vi "002_Data Graph.vi"(11 "Queue Ref In":T1={"UI"=refnum, "Message"=refnum, "Data"=refnum, "Caller"=refnum, "Name"="相对湿度计算", "Data Path"=path "", "Class Path"=path "", "SubPanel"=refnum, "Project Name"="", "MNT"="", "Title"="", "Data Source"=refnum, "Queue List"={}, "VI"=refnum, "UE"=refnum}) -> ()   [LabVIEW 2020]
doc: "000001"
uses:
  Alin/QMH/000 Module Data Type.ctl
  Alin/QMH/Queue Message.ctl
  <vilib>/Utility/miscctls.llb/LVMapReplaceAction.ctl
  70220797-d935-4723-bcfa-58572be4f9d0.vi
  <vilib>/Utility/file.llb/Read Delimited Spreadsheet (string).vi
  <vilib>/Utility/file.llb/Write Delimited Spreadsheet (string).vi
panel:
  out "字符串":string="功率电流密度曲线"
  in  "Panel Show":bool
  in  "Hide Data":bool
  in  "Hide Lable":bool
  in  "Data Select":bool
  in  "Panel Change":bool
  in  "Array":T2(array[cluster]) {"Data" format="%#.3f"}
  in  "XY":cluster{cluster{"Time":timestamp, sgl}[]}[](graph)
  in  "滑动杆":u8(slide) scale=0.0..100.0
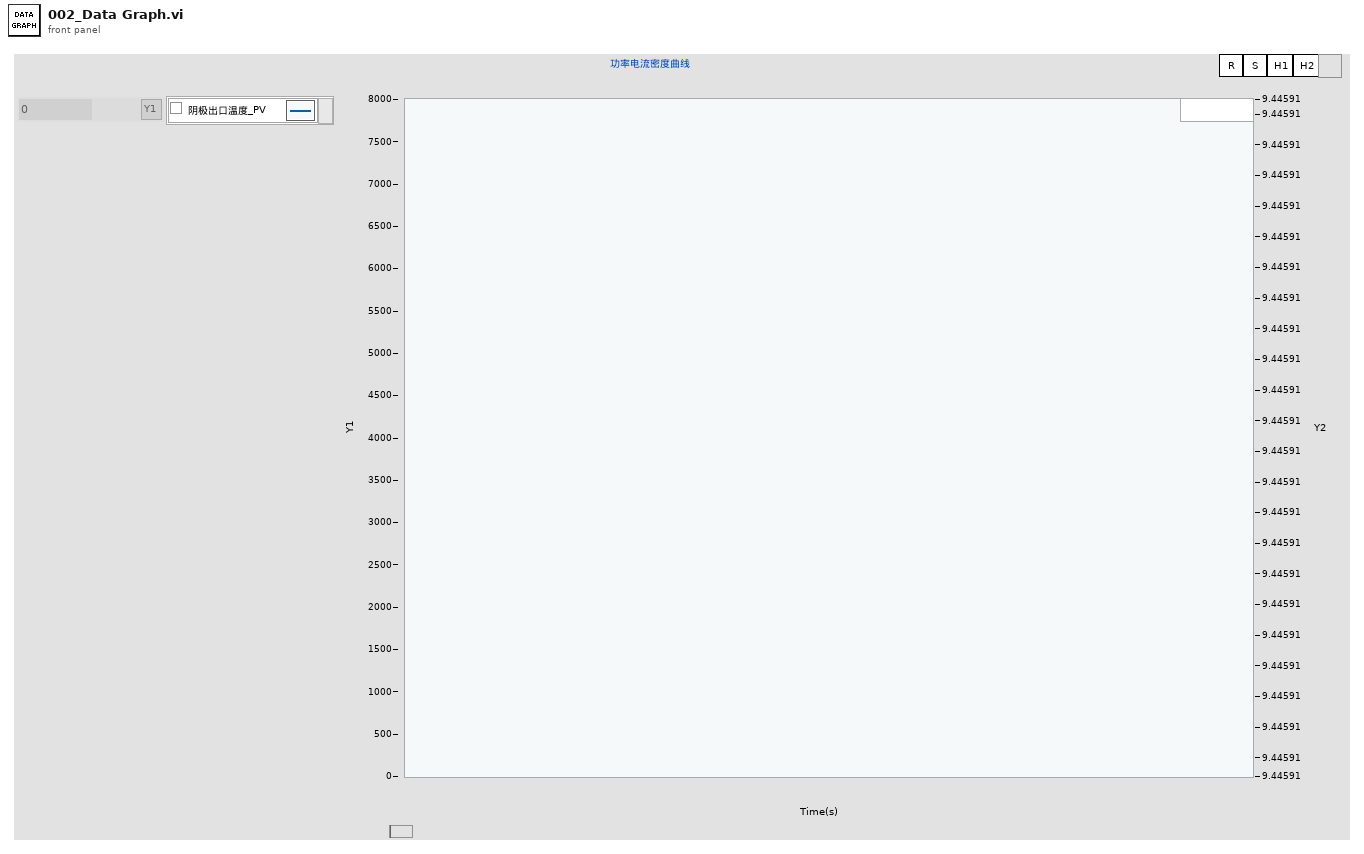
[diagram p1: front panel]
types:
  T1 = typedef "000 Module Data Type.ctl" = cluster{"UI":refnum<queue>, "Message":refnum<queue>, "Data":refnum<queue>, "Caller":refnum<queue>, "Name":string, "Data Path":path, "Class Path":path, "SubPanel":refnum<vi>, "Project Name":string, "MNT":string, "Title":string, "Data Source":refnum<queue>, "Queue List":map{string, refnum<queue>}, "VI":refnum<vi>, "UE":refnum<user-event>}
  T2 = cluster{"Identifier":string, "Data":dbl, "Unit":string, "Y":bool}[]
  T3 = cluster{"Queue Ref":T1, "Identifiers":string[], "XY":map{string, cluster{cluster{"Time":timestamp, sgl}[]}}, "Save Judge":cluster{"Time":cluster{"Name":string, "Delay":u64, "Number":u32, "Last Time":u64}[]}, "Delay":cluster{"Count Time(ms)":u32, "Delay Time(ms)":u32, "Next":string}}
  T4 = typedef "LVMapReplaceAction.ctl" = enum32{"Modify Entry only if found", "Add or Modify Entry", "Delete Entry"}
  T5 = cluster{"Name":string, "Delay":u64, "Number":u32, "Last Time":u64}[]
  T6 = cluster{"Name":string, "Delay":u64, "Number":u32, "Last Time":u64}
  T7 = typedef "SDQ Data Type.ctl" = cluster{"CAN Length":string, "CAN Name":string, "CAN ID":string, "CAN Type":string, "Test Item":string, "Byte Order":string, "Instruction":string, "Control Type":string, "Group":string, "Offset":dbl, "Coefficient":dbl, "Write Enable":bool, "Lable Type":string, "Key?":string, "Set Value":string, "Upper":dbl, "Lower":dbl, "Unit":string, "Formula":string, "Test Item Type":string, "Length":i32, "Address":string, "Name":string, "Identifier":string, "Data Type":string, "Enumerate?":string, "Enumerate List":string, "Data":string, "Source":string}
  T8 = cluster{"Identifier":string, "Data":dbl, "Unit":string, "Y":bool}
  T9 = map{string, cluster{cluster{"Time":timestamp, sgl}[]}}
  T10 = cluster{"Data Out":cluster{"Time":timestamp, sgl}[]}
  T11 = typedef "eventvkey.ctl" = enum16{"ASCII", "Enter", "Return", "Shift", "Ctrl", "Alt", "Cmd", "Opt", "Caps", "NumLock", "Clear", "Break", "Up", "Down", "Left", "Right", "Insert", "Delete", "Home", "End", "PageUp", "PageDown", "Escape", "Help", "Pause", "ScrollLock", "F1", "F2", "F3", "F4", "F5", "F6", "F7", "F8", "F9", "F10", "F11", "F12", "F13", "F14", "F15", "F16", "F17", "F18", "F19", "F20", "F21", "F22", "F23", "F24", "Play", "VolumeUp", "VolumeDown", "Mute", "Two Byte Char"}
  T12 = cluster{"Shift":bool, "Ctrl":bool, "Alt":bool, "Cmd":bool, "Opt":bool}
  T13 = typedef "LVPoint32TypeDef.ctl" = cluster{"Horizontal":i32, "Vertical":i32}
  T14 = cluster{"Queue Ref":T1, "Identifiers":string[], "XY":refnum<vi>, "Array":refnum<vi>, "Spliter":refnum<vi>}
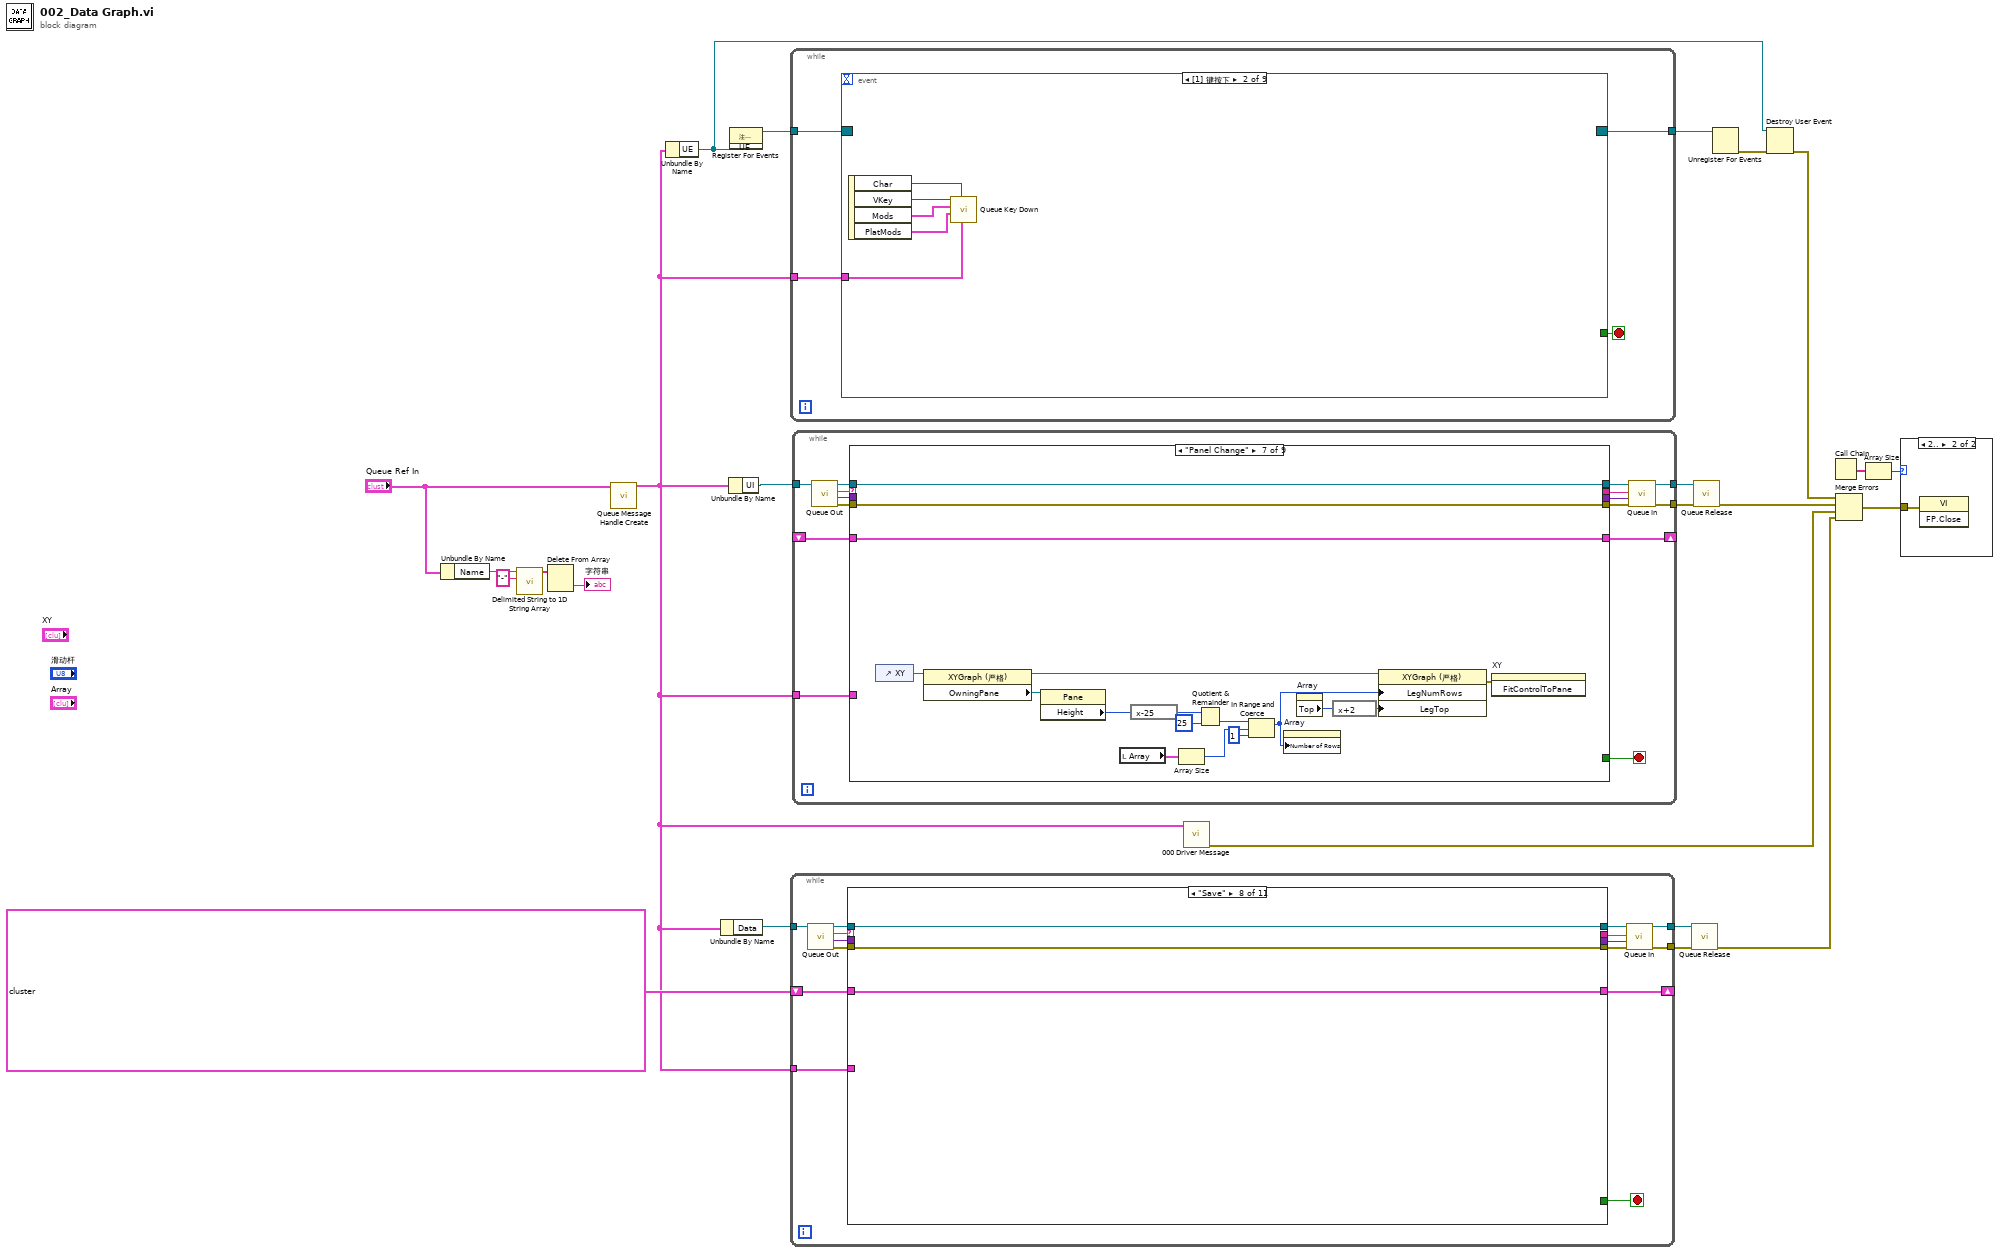
[diagram p0: block diagram]
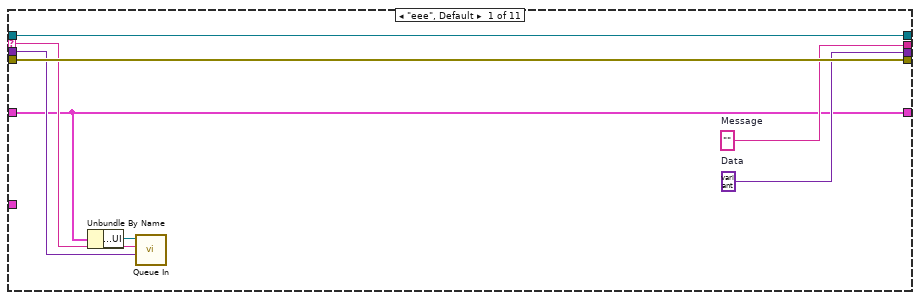
[diagram p2: hidden frame]
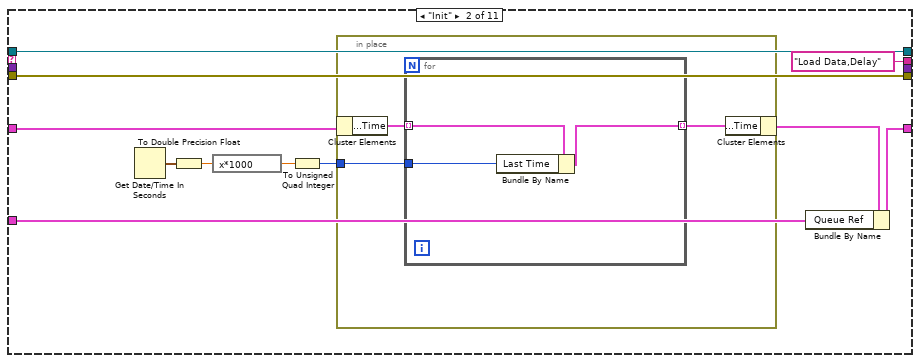
[diagram p3: hidden frame]
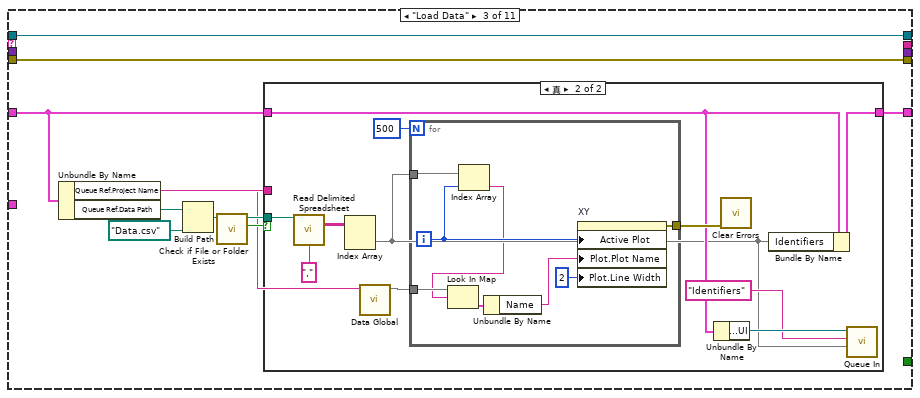
[diagram p4: hidden frame]
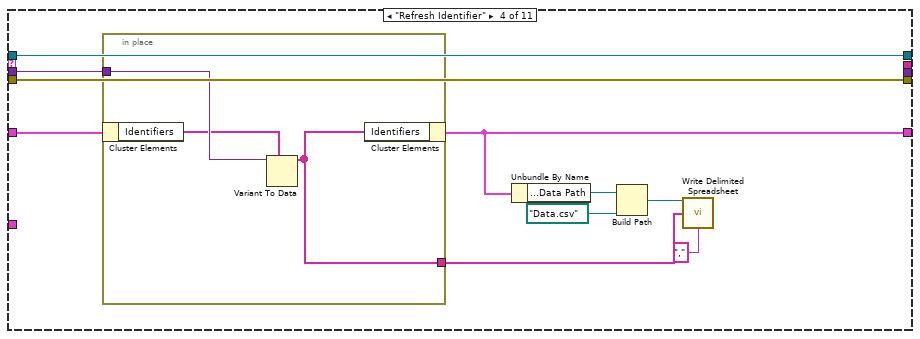
[diagram p6: hidden frame]
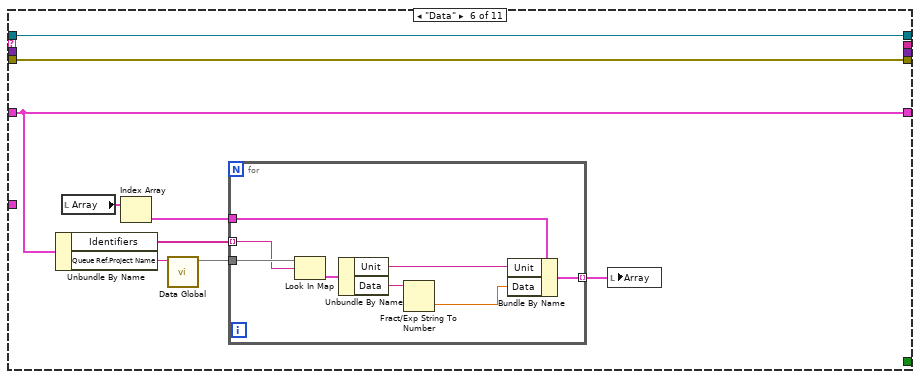
[diagram p8: hidden frame]
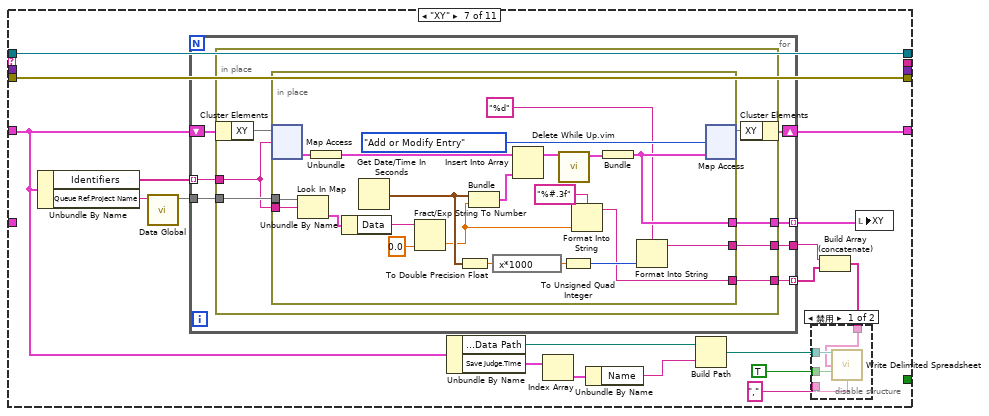
[diagram p9: hidden frame]
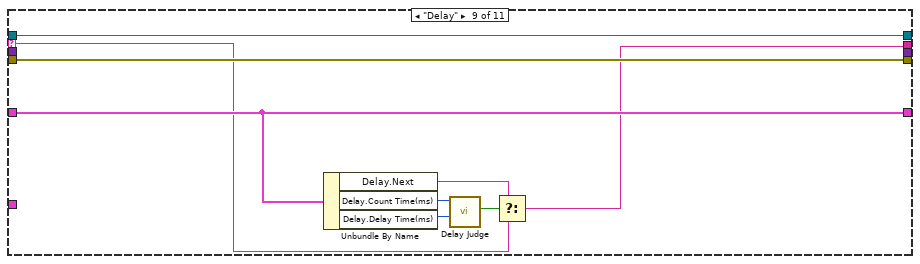
[diagram p11: hidden frame]
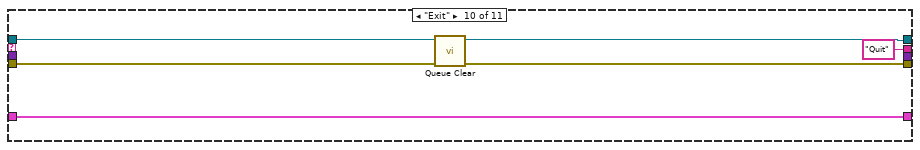
[diagram p12: hidden frame]
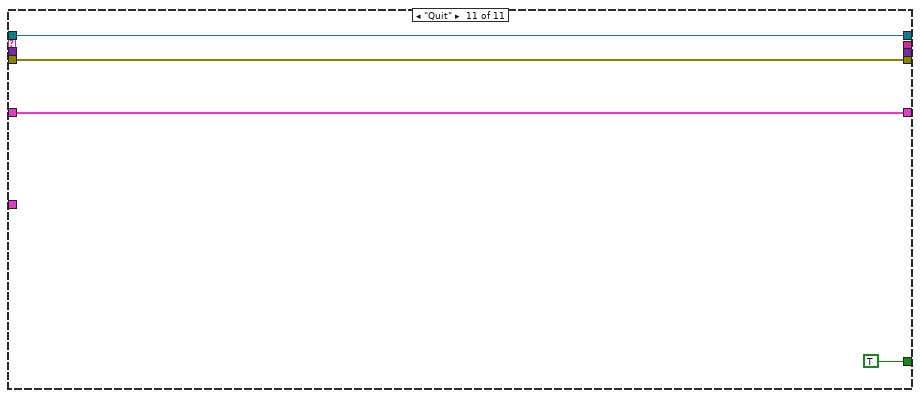
[diagram p13: hidden frame]
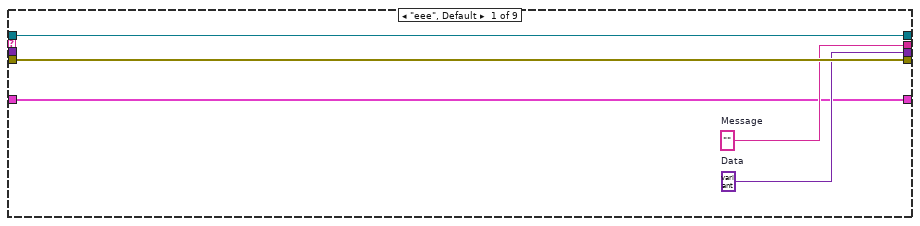
[diagram p15: hidden frame]
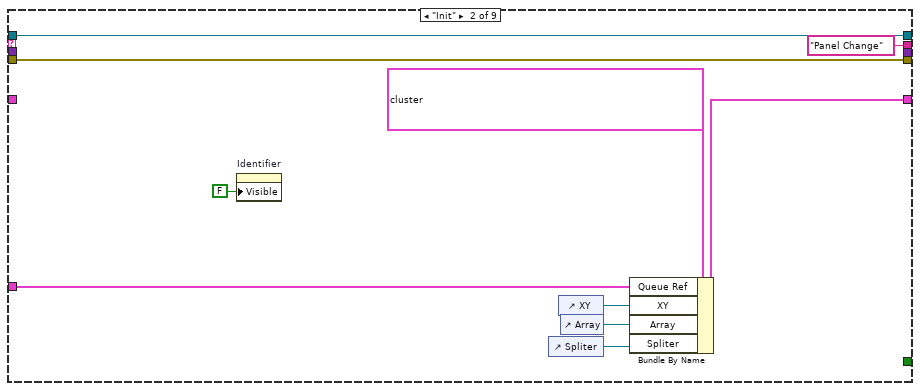
[diagram p16: hidden frame]
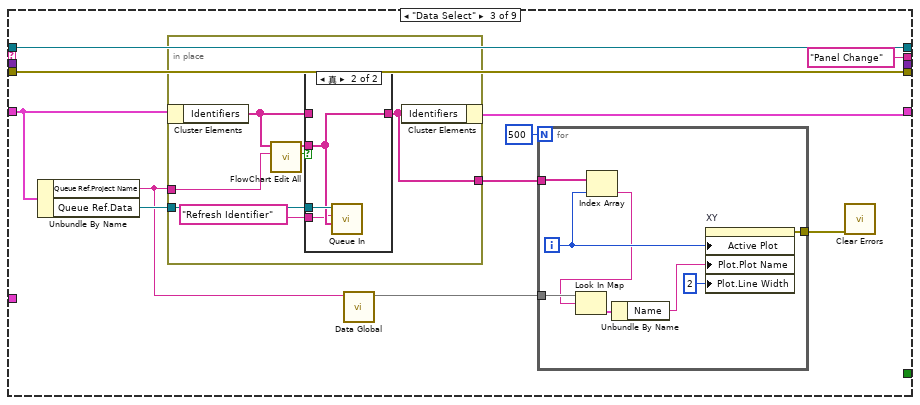
[diagram p17: hidden frame]
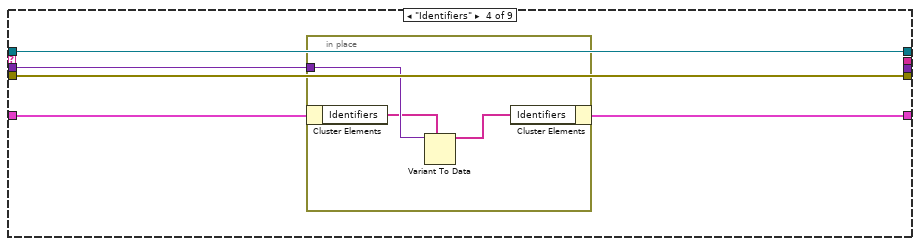
[diagram p19: hidden frame]
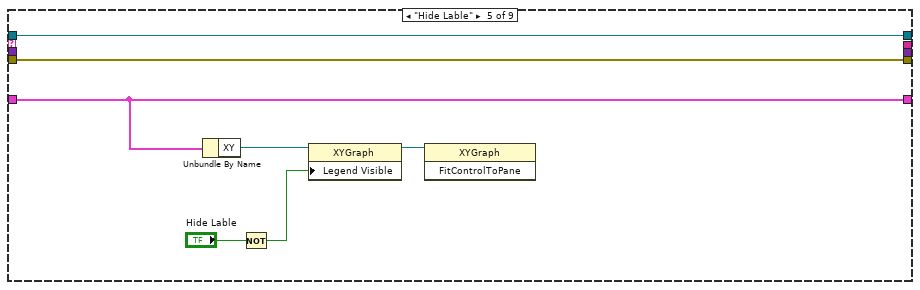
[diagram p20: hidden frame]
diagram:
  n1 = Unbundle By Name("Queue Ref In") -> ("Name"=w6:string)
  n2 = call <vilib>:"Delimited String to 1D String Array.vi"("delimiter"="-", "delimited string"=w6) -> ("string array"=w4:string[])  [unwired: 9 in]
  n3 = Delete From Array(array=w4) -> (deleted portion=→"字符串":string)  [unwired: 2 in, 1 out]
  n4 = call "Queue Message Handle Create.vi"("Queue Ref In"="Queue Ref In") -> ("Queue Ref Out"=w2:T1)  [unwired: 9 in, 1 out]
  n5 = Unbundle By Name(w2) -> ("UE"=w1:refnum<user-event>)
  n6 = Unbundle By Name(w2) -> ("Data"=w22:refnum<queue>)
  n7 = Unbundle By Name(w2) -> ("UI"=w14:refnum<queue>)
  n8 = register-events(w1) -> (reference out=w9:refnum<event-registration>)  [unwired: 2 in, 1 out]
  n9 = while {
    tunnel: w22 -> [w35]
    tunnel: [w32] -> w20
    tunnel: [w31] -> w21
    shift-right: [w27] -> _
    shift-left: T3 {"Queue Ref"={"UI"=refnum, "Message"=refnum, "Data"=refnum, "Caller"=refnum, "Name"="相对湿度计算", "Data Path"=path "", "Class Path"=path "", "SubPanel"=refnum, "Project Name"="", "MNT"="", "Title"="", "Data Source"=refnum, "Queue List"={}, "VI"=refnum, "UE"=refnum}, "Identifiers"=[], "XY"={}, "Save Judge"={"Time"=[{"Name"="Fast.csv", "Delay"=200, "Number"=0, "Last Time"=0}, {"Name"="Middle.csv", "Delay"=1000, "Number"=0, "Last Time"=0}, {"Name"="Middle.csv", "Delay"=10000, "Number"=0, "Last Time"=0}]}, "Delay"={"Count Time(ms)"=50, "Delay Time(ms)"=50, "Next"="Data,XY,Save,Delay"}} -> [w26]
    tunnel: w2 -> [w25]
    stop <- w39 stop-if-true
    n10 = call "Queue Out.vi"("Queue In"=w35) -> ("error out"=w38:errorcluster, "Data"=w36:variant, "Message"=w37:string, "Queue Out"=w34:refnum<queue>)  [unwired: 6 in, 1 out]
    n11 = case shown="\"Save\"" w37 {
      selector: w37 -> [w43 _ _ _ _ _ _ _ w190 _ _]
      tunnel: w34 -> [w47 w58 w74 w105 w111 w120 w146 w188 w197 w202 w206]
      tunnel: w38 -> [w46 w57 w73 w104 w110 w119 w145 w187 w196 w200 w207]
      tunnel: [w47 w58 w74 w105 w111 w120 w146 w188 w197 w201 w206] -> w33
      tunnel: [w46 w57 w73 w104 w110 w119 w145 w187 w196 w199 w207] -> w30
      tunnel: [w45 "Load Data,Delay" ("Message") _ _ _ _ _ _ w189 "Quit" _] -> w29
      tunnel: [_ _ _ _ _ _ _ _ _ _ TRUE] -> w39
      tunnel: [w44 _ _ _ _ _ _ _ _ _ _] -> w28
      tunnel: w36 -> [w42 _ _ w102 _ _ _ _ _ _ _]
      tunnel: [w41 w56 w67 w101 w109 w112 w144 w186 w191 w198 w204] -> w27
      tunnel: w26 -> [w41 w55 w68 w103 w109 w112 w132 w186 w191 w198 w204]
      tunnel: w25 -> [_ w48 _ _ _ _ _ _ _ _ _]
      frame "eee", Default {
        w44 = variant  # Data
        w45 = ""  # Message
        n12 = Unbundle By Name(w41) -> ("Queue Ref.UI"=w40:refnum<queue>)
        n13 = call "Queue In.vi"("Data"=w42, "Message"=w43, "Queue In"=w40) -> ()  [unwired: 7 in, 2 out]
      }
      frame "Init" {
        n14 = Get Date/Time In Seconds() -> (seconds since 1Jan1904=w53:timestamp)
        n15 = To Double Precision Float(number=w53) -> (double precision float=w52:dbl)
        n16 = expression code="x*1000"(w52) -> (w51:dbl)
        n17 = To Unsigned Quad Integer(1:w51) -> (0:w50:u64)
        n18 = in-place {
          in-place-border: w50 -> [w60]
          n19 = in-place-cluster #1(w55) -> ("Save Judge.Time"=w61:T5)
          n20 = for {
            tunnel: w61 -> [w64] mode=indexing
            tunnel: w60 -> [w63]
            tunnel: [w62] -> w59 mode=indexing
            n21 = Bundle By Name(cluster=w64, "Last Time"=w63) -> (w62:T6)
          }
          n22 = in-place-cluster #1("Save Judge.Time"=w59) -> (w54:T3)
        }
        n23 = Bundle By Name(cluster=w54, "Queue Ref"=w48) -> (w56:T3)
      }
      frame "Load Data" {
        n24 = Unbundle By Name(w68) -> ("Queue Ref.Project Name"=w65:string, "Queue Ref.Data Path"=w72:path)
        n25 = Build Path(base path=w72, name or relative path=path "Data.csv" ("名称或相对路径")) -> (appended path=w70:path)
        n26 = call <vilib>:"Check if File or Folder Exists.vi"("path"=w70) -> ("file or folder exists?"=w66:bool, "dup path"=w69:path)  [unwired: 8 in, 1 out]
        n27 = case shown="真" w66 {
          tunnel: w69 -> [_ w86]
          tunnel: w68 -> [w75 w77]
          tunnel: [w75 w84] -> w67
          tunnel: w65 -> [_ w83]
          frame False {
          }
          frame True {
            n28 = call-poly <vilib>:"Read Delimited Spreadsheet.vi"("file path (dialog if empty)"=w86, "delimiter (\\t)"="," ("delimiter (\\t)")) -> ("all rows"=w87:string[][])  [unwired: 8 in, 5 out]
            n29 = Index Array(array=w87) -> (element=w76:string[])  [unwired: 2 in]
            n30 = call "Data Global.vi"("Name"=w83) -> ("Data Out"=w82:map{string, T7})  [unwired: 7 in, 3 out]
            n31 = for {
              N: 500 -> [_]
              tunnel: [w95] -> w81
              tunnel: w82 -> [w93]
              tunnel: w76 -> [w91]
              i -> [w90]
              n32 = Index Array(array=w91, index=w90) -> (element=w89:string)
              n33 = Look In Map(map=w93, key=w89) -> (value=w94:T7)  [unwired: 1 in, 1 out]
              n34 = Unbundle By Name(w94) -> ("Name"=w92:string)
              n35 = property on="XY" class="XYGraph (严格)"("Active Plot"=w90, "Plot.Plot Name"=w92, "Plot.Line Width"=u8 2 ("曲线.线条宽度")) -> (error out=w95:errorcluster)  [unwired: 2 in, 1 out]
            }
            n36 = Unbundle By Name(w77) -> ("Queue Ref.UI"=w79:refnum<queue>)
            n37 = call <vilib>:"Clear Errors.vi"("error in (no error)"=w81) -> ()  [unwired: 5 in, 2 out]
            n38 = Bundle By Name(cluster=w77, "Identifiers"=w76) -> (w84:T3)
            n39 = call "Queue In.vi"("Data"=w76, "Message"="Identifiers", "Queue In"=w79) -> ()  [unwired: 7 in, 2 out]
          }
        }
      }
      frame "Refresh Identifier" {
        n40 = in-place {
          in-place-border: w102 -> [w108]
          in-place-border: [w106] -> w96
          n41 = in-place-cluster #2(w103) -> ("Identifiers"=w107:string[])
          n42 = Variant To Data(type=w107, Variant=w108) -> (data=w106:string[])  [unwired: 1 in, 1 out]
          n43 = in-place-cluster #2("Identifiers"=w106) -> (w101:T3)
        }
        n44 = Unbundle By Name(w101) -> ("Queue Ref.Data Path"=w100:path)
        n45 = Build Path(base path=w100, name or relative path=path "Data.csv" ("名称或相对路径")) -> (appended path=w99:path)
        n46 = call-poly <vilib>:"Write Delimited Spreadsheet.vi"("file path (dialog if empty)"=w99, "1D data"=w96, "delimiter (\\t)"="," ("delimiter (\\t)")) -> ()  [unwired: 11 in, 2 out]
      }
      frame "Data Select" {
      }
      frame "Data" {
        n47 = Unbundle By Name(w112) -> ("Identifiers"=w116:string[], "Queue Ref.Project Name"=w118:string)
        n48 = local read "Array"() -> (w115:T2)
        n49 = Index Array(array=w115) -> (element=w114:T8)  [unwired: 1 in]
        n50 = call "Data Global.vi"("Name"=w118) -> ("Data Out"=w117:map{string, T7})  [unwired: 7 in, 3 out]
        n51 = for {
          tunnel: w117 -> [w128]
          tunnel: w116 -> [w121] mode=indexing
          tunnel: w114 -> [w127]
          tunnel: [w124] -> w113 mode=indexing
          n52 = Look In Map(map=w128, key=w121) -> (value=w126:T7)  [unwired: 1 in, 1 out]
          n53 = Unbundle By Name(w126) -> ("Unit"=w125:string, "Data"=w123:string)
          n54 = Fract/Exp String To Number(string=w123) -> (number=w122:dbl)  [unwired: 3 in, 1 out]
          n55 = Bundle By Name(cluster=w127, "Unit"=w125, "Data"=w122) -> (w124:T8)
        }
        n56 = local write "Array"(w113) -> ()
      }
      frame "XY" {
        n57 = Unbundle By Name(w132) -> ("Identifiers"=w143:string[], "Queue Ref.Project Name"=w142:string)
        n58 = call "Data Global.vi"("Name"=w142) -> ("Data Out"=w141:map{string, T7})  [unwired: 7 in, 3 out]
        n59 = for {
          shift-right: [w156] -> w144
          shift-left: w132 -> [w157]
          tunnel: w143 -> [w155] mode=indexing
          tunnel: w141 -> [w154]
          tunnel: [w153] -> w140 mode=indexing
          tunnel: [w152] -> w131
          tunnel: [w151] -> w130 mode=indexing
          n60 = in-place {
            in-place-border: w155 -> [w160]
            in-place-border: w154 -> [w162]
            in-place-border: [w161] -> w153
            in-place-border: [w159] -> w152
            in-place-border: [w158] -> w151
            n61 = in-place-cluster #3(w157) -> ("XY"=w164:T9)
            n62 = in-place {
              in-place-border: w162 -> [w179]
              in-place-border: w160 -> [w177]
              in-place-border: [w176] -> w161
              in-place-border: [w168] -> w159
              in-place-border: [w167] -> w158
              n63 = in-place-map #4(w164, w160) -> (w184:cluster{cluster{"Time":timestamp, sgl}[]})  [unwired: 1 in, 1 out]
              n64 = Look In Map(map=w179, key=w177) -> (value=w181:T7)  [unwired: 1 in, 1 out]
              n65 = Unbundle(w184) -> (w183:cluster{"Time":timestamp, sgl}[])
              n66 = Unbundle By Name(w181) -> ("Data"=w180:string)
              n67 = Get Date/Time In Seconds() -> (seconds since 1Jan1904=w173:timestamp)
              n68 = Fract/Exp String To Number(string=w180, default (0 dbl)=sgl 0.0 ("默认(0 DBL)")) -> (number=w169:sgl)  [unwired: 2 in, 1 out]
              n69 = To Double Precision Float(number=w173) -> (double precision float=w175:dbl)
              n70 = Bundle("seconds since 1Jan1904"=w173, w169) -> (w182:cluster{"seconds since 1Jan1904":timestamp, sgl})  [unwired: 1 in]
              n71 = expression code="x*1000"(w175) -> (w174:dbl)
              n72 = Insert Into Array(array=w183, new element=w182) -> (w166:cluster{"Time":timestamp, sgl}[])  [unwired: 1 in]
              n73 = call "Delete While Up.vim"("Data In"=w166) -> ("Data Out"=w165:cluster{"Time":timestamp, sgl}[])  [unwired: 10 in]
              n74 = To Unsigned Quad Integer(1:w174) -> (0:w171:u64)
              n75 = Format Into String(format string="%#.3f" ("格式字符串"), w169) -> (resulting string=w167:string)  [unwired: 2 in, 1 out]
              n76 = Bundle("Data Out"=w165) -> (w176:T10)  [unwired: 1 in]
              n77 = Format Into String(format string="%d" ("格式字符串"), w171) -> (resulting string=w168:string)  [unwired: 2 in, 1 out]
              n78 = in-place-map #4(w176, LVMapReplaceAction."Add or Modify Entry" ("操作")) -> (w163:T9)  [unwired: 2 out]
            }
            n79 = in-place-cluster #3("XY"=w163) -> (w156:T3)
          }
        }
        n80 = Unbundle By Name(w132) -> ("Queue Ref.Data Path"=w137:path, "Save Judge.Time"=w139:T5)
        n81 = Index Array(array=w139) -> (element=w138:T6)  [unwired: 1 in]
        n82 = Unbundle By Name(w138) -> ("Name"=w136:string)
        n83 = Build Path(base path=w137, name or relative path=w136) -> (appended path=w135:path)
        n84 = Build Array (concatenate)(w131, w130) -> (w129:string[])
        n85 = disable-structure shown="禁用" {
          disable-tunnel: w135 -> [w150 _]
          disable-tunnel: TRUE ("append to file? (new file:F)") -> [w149 _]
          disable-tunnel: "," ("delimiter (\\t)") -> [w148 _]
          disable-tunnel: w129 -> [w147 _]
          frame Disabled {
            n86 = call-poly <vilib>:"Write Delimited Spreadsheet.vi"("file path (dialog if empty)"=w150, "1D data"=w147, "append to file? (new file:F)"=w149, "delimiter (\\t)"=w148) -> ()  [unwired: 10 in, 2 out]
          }
          frame Enabled {
          }
        }
        n87 = local write "XY"(w140) -> ()
      }
      frame "Save" {
      }
      frame "Delay" {
        n88 = Unbundle By Name(w191) -> ("Delay.Next"=w192:string, "Delay.Count Time(ms)"=w195:u32, "Delay.Delay Time(ms)"=w194:u32)
        n89 = call "Delay Judge.vi"("Delay Time(ms)"=w194, "Count Time(ms)"=w195) -> ("Time Out?"=w193:bool)  [unwired: 5 in, 4 out]
        n90 = Select(t=w192, s=w193, f=w190) -> (s? t:f=w189:string)
      }
      frame "Exit" {
        n91 = call "Queue Clear.vi"("error in (no error)"=w200, "Queue In"=w202) -> ("error out"=w199:errorcluster, "Queue Out"=w201:refnum<queue>)  [unwired: 8 in]
      }
      frame "Quit" {
      }
    }
    n92 = call "Queue In.vi"("error in (no error)"=w30, "Data"=w28, "Message"=w29, "Queue In"=w33) -> ("error out"=w31:errorcluster, "Queue Out"=w32:refnum<queue>)  [unwired: 6 in]
  }
  n93 = while {
    tunnel: w9 -> [w211]
    tunnel: [w209] -> w10
    tunnel: w2 -> [w208]
    stop <- w210 stop-if-true
    n94 = event shown="[1] 键按下" {
      selector: w211 -> [_ _ _ _ _ _ _ _ _]
      dyn-events: [_ _ _ _ _ _ _ _ _] -> w209
      timeout: _ -> [_ _ _ _ _ _ _ _ _]
      tunnel: [_ _ _ w223 _ _ _ _ _] -> w210
      tunnel: w208 -> [w214 w218 w222 _ w228 _ w242 _ w260]
      event Timeout {
        n95 = event-data() -> ()  [unwired: 1 in, 1 out]
        n96 = Unbundle By Name(w214) -> ("Data"=w213:refnum<queue>)
        n97 = call "Queue In.vi"("Message"="Data", "Queue In"=w213) -> ()  [unwired: 8 in, 2 out]
      }
      event Key Down {
        n98 = event-data() -> ("Char"=w219:i16, "VKey"=w217:T11, "Mods"=w216:cluster{"Num Pad":bool, "Menu Key":bool}, "PlatMods"=w215:T12)  [unwired: 1 in]
        n99 = call "Queue Key Down.vi"("Queue Ref Out"=w218, "C"=w219, "Platform Key"=w215, "Group Key"=w216, "V Key"=w217) -> ()  [unwired: 6 in, 1 out]
      }
      event Panel Resize {
        n100 = event-data() -> ()  [unwired: 1 in, 1 out]
        n101 = Unbundle By Name(w222) -> ("UI"=w221:refnum<queue>)
        n102 = call "Queue In.vi"("Message"="Panel Change", "Queue In"=w221) -> ()  [unwired: 8 in, 2 out]
      }
      event User Event {
        n103 = event-data() -> ("Message"=w225:string)  [unwired: 1 in]
        n104 = Equal?(x=w225, y="Exit") -> (x = y?=w223:bool)
      }
      event Panel Close? {
        n105 = event-data() -> ()  [unwired: 1 in, 1 out]
        n106 = Call Chain() -> (call chain=w230:string[])
        n107 = Array Size(array=w230) -> (size(s)=w229:i32)
        n108 = case shown="1" w229 {
          tunnel: w228 -> [w234 w237]
          tunnel: [w233 w236] -> w227
          tunnel: ["Panel Hidden" ("Message") "Exit Prepare" ("Message")] -> w226
          frame 2, Default {
            n109 = Unbundle By Name(w234) -> ("Message"=w233:refnum<queue>)
          }
          frame 1 {
            n110 = Unbundle By Name(w237) -> ("Message"=w236:refnum<queue>)
          }
        }
        n111 = call "Queue In.vi"("Message"=w226, "Queue In"=w227) -> ()  [unwired: 8 in, 2 out]
        n112 = event-data("Discard?"=TRUE ("放弃？")) -> ()  [unwired: 1 in, 1 out]
      }
      event "XY": Mouse Wheel {
        n113 = event-data() -> ("CtlRef"=w241:refnum<vi>)  [unwired: 1 in]
        n114 = property class="XYGraph (严格)"(reference=w241) -> ("LegScrollPos"=w240:u32, "LegNumRows"=w238:u32)  [unwired: 1 in, 2 out]
        n115 = Build Array(w240) -> (w239:u32[])
        n116 = property on="Array" class="Arr (严格)"("Index Values"=w239, "Number of Rows"=w238) -> ()  [unwired: 2 in, 2 out]
      }
      event "Data Select", "Panel Change", "Hide Lable", "Hide Data": Value Change {
        n117 = event-data() -> ("CtlRef"=w244:refnum<vi>)  [unwired: 1 in]
        n118 = Unbundle By Name(w242) -> ("UI"=w245:refnum<queue>)
        n119 = property class="Bool"(reference=w244) -> ("Label.Text"=w243:string)  [unwired: 1 in, 2 out]
        n120 = call "Queue In.vi"("Message"=w243, "Queue In"=w245) -> ()  [unwired: 8 in, 2 out]
        n121 = case shown="\"Panel Change\"" w243 {
          tunnel: w242 -> [_ w248]
          frame "假", Default {
          }
          frame "Panel Change" {
            n122 = Unbundle By Name(w248) -> ("Data"=w247:refnum<queue>)
            n123 = call "Queue In.vi"("Message"="Load Data", "Queue In"=w247) -> ()  [unwired: 8 in, 2 out]
          }
        }
      }
      event "XY": Mouse Move {
        n124 = event-data() -> ("CtlRef"=w250:refnum<vi>, "Coords"=w249:T13)  [unwired: 1 in]
        n125 = disable-structure shown="禁用" {
          disable-tunnel: w250 -> [w256 _]
          disable-tunnel: w249 -> [w255 _]
          frame Disabled {
            n126 = invoke class="XYGraph (严格)" method="Map Coords To XY"(reference=w256, "Coords"=w255) -> (reference out=w253:refnum<vi>, "XY"=w254:cluster{"X":dbl, "Y":dbl})  [unwired: 5 in, 5 out]
            n127 = Unbundle By Name(w254) -> ("X"=w251:dbl)
            n128 = property class="XYGraph (严格)"(reference=w253, "Active Cursor"=u32 0 ("活动游标"), "Cursor.Cursor X"=w251) -> ()  [unwired: 1 in, 2 out]
          }
          frame Enabled {
          }
        }
      }
      event "Panel Show": Value Change {
        n129 = event-data() -> ("CtlRef"=w259:refnum<vi>)  [unwired: 1 in]
        n130 = Unbundle By Name(w260) -> ("Message"=w258:refnum<queue>)
        n131 = property class="Bool"(reference=w259) -> ("Label.Text"=w257:string)  [unwired: 1 in, 2 out]
        n132 = call "Queue In.vi"("Message"=w257, "Queue In"=w258) -> ()  [unwired: 8 in, 2 out]
      }
    }
  }
  n133 = while {
    tunnel: w14 -> [w271]
    tunnel: [w268] -> w12
    tunnel: [w267] -> w13
    shift-right: [w263] -> _
    shift-left: _ -> [w262]
    tunnel: w2 -> [w261]
    stop <- w275 stop-if-true
    n134 = call "Queue Out.vi"("Queue In"=w271) -> ("error out"=w274:errorcluster, "Data"=w272:variant, "Message"=w273:string, "Queue Out"=w270:refnum<queue>)  [unwired: 6 in, 1 out]
    n135 = case shown="\"Panel Change\"" w273 {
      selector: w273 -> [_ _ _ _ _ _ _ w366 _]
      tunnel: w270 -> [w280 w290 w301 w325 w335 w346 w363 w373 w379]
      tunnel: w274 -> [w279 w289 w300 w324 w334 w345 w362 w371 w380]
      tunnel: [w280 w290 w301 w325 w335 w346 w363 w372 w379] -> w269
      tunnel: [w279 w289 w300 w324 w334 w345 w362 w370 w380] -> w266
      tunnel: [w278 "Panel Change" ("Message") "Panel Change" ("Message") _ _ _ _ "Quit" _] -> w265
      tunnel: [_ _ _ _ _ _ _ _ TRUE] -> w275
      tunnel: [w277 _ _ _ _ _ _ _ _] -> w264
      tunnel: w272 -> [_ _ _ w321 _ _ _ _ _]
      tunnel: [w276 w285 w296 w322 w333 w344 w348 w365 w377] -> w263
      tunnel: w262 -> [w276 _ w299 w323 w333 w344 w348 w365 w377]
      tunnel: w261 -> [_ w284 _ _ _ _ _ _ _]
      frame "eee", Default {
        w277 = variant  # Data
        w278 = ""  # Message
      }
      frame "Init" {
        n136 = property on="Identifier" class="Str"("Visible"=FALSE ("可见")) -> ()  [unwired: 2 in, 2 out]
        n137 = control-ref of="Spliter"() -> (w281:refnum<vi>)
        n138 = control-ref of="XY"() -> (w283:refnum<vi>)
        n139 = control-ref of="Array"() -> (w282:refnum<vi>)
        n140 = Bundle By Name(cluster=T14 {"Queue Ref"={"UI"=refnum, "Message"=refnum, "Data"=refnum, "Caller"=refnum, "Name"="相对湿度计算", "Data Path"=path "", "Class Path"=path "", "SubPanel"=refnum, "Project Name"="", "MNT"="", "Title"="", "Data Source"=refnum, "Queue List"={}, "VI"=refnum, "UE"=refnum}, "Identifiers"=[], "XY"=refnum, "Array"=refnum, "Spliter"=refnum}, "Queue Ref"=w284, "XY"=w283, "Array"=w282, "Spliter"=w281) -> (w285:T14)
      }
      frame "Data Select" {
        n141 = Unbundle By Name(w299) -> ("Queue Ref.Project Name"=w295:string, "Queue Ref.Data"=w298:refnum<queue>)
        n142 = in-place {
          in-place-border: w295 -> [w316]
          in-place-border: w298 -> [w312]
          in-place-border: [w310] -> w293
          n143 = in-place-cluster #5(w299) -> ("Identifiers"=w313:string[])
          n144 = call "FlowChart Edit All.vi"("Name"=w316, "Identifier In"=w313) -> ("OK？"=w315:bool, "Identifiers Out"=w314:string[])  [unwired: 8 in]
          n145 = case shown="真" w315 {
            tunnel: w314 -> [_ w319]
            tunnel: [w317 w319] -> w310
            tunnel: w313 -> [w317 _]
            tunnel: w312 -> [_ w320]
            tunnel: "Refresh Identifier" ("Message") -> [_ w318]
            frame False {
            }
            frame True {
              n146 = call "Queue In.vi"("Data"=w319, "Message"=w318, "Queue In"=w320) -> ()  [unwired: 7 in, 2 out]
            }
          }
          n147 = in-place-cluster #5("Identifiers"=w310) -> (w296:T14)
        }
        n148 = call "Data Global.vi"("Name"=w295) -> ("Data Out"=w294:map{string, T7})  [unwired: 7 in, 3 out]
        n149 = for {
          N: 500 -> [_]
          tunnel: [w309] -> w297
          tunnel: w294 -> [w307]
          tunnel: w293 -> [w305]
          i -> [w304]
          n150 = Index Array(array=w305, index=w304) -> (element=w303:string)
          n151 = Look In Map(map=w307, key=w303) -> (value=w308:T7)  [unwired: 1 in, 1 out]
          n152 = Unbundle By Name(w308) -> ("Name"=w306:string)
          n153 = property on="XY" class="XYGraph (严格)"("Active Plot"=w304, "Plot.Plot Name"=w306, "Plot.Line Width"=u8 2 ("曲线.线条宽度")) -> (error out=w309:errorcluster)  [unwired: 2 in, 1 out]
        }
        n154 = call <vilib>:"Clear Errors.vi"("error in (no error)"=w297) -> ()  [unwired: 5 in, 2 out]
      }
      frame "Identifiers" {
        n155 = in-place {
          in-place-border: w321 -> [w328]
          n156 = in-place-cluster #6(w323) -> ("Identifiers"=w327:string[])
          n157 = Variant To Data(type=w327, Variant=w328) -> (data=w326:string[])  [unwired: 1 in, 1 out]
          n158 = in-place-cluster #6("Identifiers"=w326) -> (w322:T14)
        }
      }
      frame "Hide Lable" {
        n159 = Unbundle By Name(w333) -> ("XY"=w332:refnum<vi>)
        n160 = Not(x="Hide Lable") -> (.not. x?=w330:bool)
        n161 = property class="XYGraph"(reference=w332, "Legend Visible"=w330) -> (reference out=w329:refnum<vi>)  [unwired: 1 in, 1 out]
        n162 = invoke class="XYGraph" method="FitControlToPane"(reference=w329) -> ()  [unwired: 2 in, 3 out]
      }
      frame "Hide Data" {
        n163 = Unbundle By Name(w344) -> ("Spliter"=w341:refnum<vi>, "Array"=w343:refnum<vi>)
        n164 = Not(x="Hide Data") -> (.not. x?=w340:bool)
        n165 = property class="Arr (严格)"(reference=w343, "Visible"=w340) -> (error out=w336:errorcluster)  [unwired: 1 in, 1 out]
        n166 = Select(t=148 ("分隔栏位置"), s=w340, f=4 ("分隔栏位置")) -> (s? t:f=w337:i32)
        n167 = property class="Splitter"(reference=w341, error in=w336, "Position"=w337) -> ()  [unwired: 2 out]
      }
      frame "Panel Change" {
        n168 = control-ref of="XY"() -> (w361:refnum<vi>)
        n169 = property class="XYGraph (严格)"(reference=w361) -> (reference out=w359:refnum<vi>, "OwningPane"=w360:refnum<vi>)  [unwired: 1 in, 1 out]
        n170 = property class="Pane"(reference=w360) -> ("Height"=w358:u32)  [unwired: 1 in, 2 out]
        n171 = local read "Array"() -> (w357:T2)
        n172 = expression code="x-25"(w358) -> (w349:u32)
        n173 = Array Size(array=w357) -> (size(s)=w356:i32)
        n174 = Quotient & Remainder(x=w349, y=u32 25) -> (floor(x/y)=w355:u32)  [unwired: 1 out]
        n175 = In Range and Coerce(upper limit=w355, x=w356, lower limit=u32 1 ("下限")) -> (coerced(x)=w354:u32)  [unwired: 1 out]
        n176 = property on="Array" class="Arr (严格)"("Number of Rows"=w354) -> ()  [unwired: 2 in, 2 out]
        n177 = property on="Array" class="Arr (严格)"() -> ("Top"=w351:i32)  [unwired: 2 in, 2 out]
        n178 = expression code="x+2"(w351) -> (w350:i32)
        n179 = property class="XYGraph (严格)"(reference=w359, "LegNumRows"=w354, "LegTop"=w350) -> (error out=w347:errorcluster)  [unwired: 1 in, 1 out]
        n180 = invoke on="XY" class="XYGraph (严格)" method="FitControlToPane"(error in=w347) -> ()  [unwired: 2 in, 3 out]
      }
      frame "Exit" {
        n181 = Unbundle By Name(w365) -> ("Queue Ref.UE"=w364:refnum<user-event>, "Queue Ref.Message"=w369:refnum<queue>, "Queue Ref.Data"=w368:refnum<queue>)
        n182 = Build Array(w369, w368) -> (w367:refnum<queue>[])
        n183 = Generate User Event(user event=w364, event data cluster=w366) -> ()  [unwired: 2 in, 2 out]
        n184 = for {
          tunnel: w367 -> [w376] mode=indexing
          tunnel: w366 -> [w375]
          n185 = call "Queue In.vi"("Message"=w375, "Queue In"=w376) -> ()  [unwired: 8 in, 2 out]
        }
        n186 = call "Queue Clear.vi"("error in (no error)"=w371, "Queue In"=w373) -> ("error out"=w370:errorcluster, "Queue Out"=w372:refnum<queue>)  [unwired: 8 in]
      }
      frame "Quit" {
      }
    }
    n187 = call "Queue In.vi"("error in (no error)"=w266, "Data"=w264, "Message"=w265, "Queue In"=w269) -> ("error out"=w267:errorcluster, "Queue Out"=w268:refnum<queue>)  [unwired: 6 in]
  }
  n188 = call "000 Driver Message.vi"("Queue In"=w2) -> ("error out"=w24:errorcluster)  [unwired: 8 in, 2 out]
  n189 = call "Queue Release.vi"("error in (no error)"=w21, "Queue In"=w20) -> ("error out"=w23:errorcluster)  [unwired: 9 in]
  n190 = call "Queue Release.vi"("error in (no error)"=w13, "Queue In"=w12) -> ("error out"=w16:errorcluster)  [unwired: 9 in]
  n191 = Unregister For Events(event registration refnum=w10) -> (error out=w11:errorcluster)  [unwired: 1 in]
  n192 = Destroy User Event(user event=w1, error in=w11) -> (error out=w15:errorcluster)
  n193 = Call Chain() -> (call chain=w18:string[])
  n194 = Merge Errors(w15, w16, w24, w23) -> (w17:errorcluster)
  n195 = Array Size(array=w18) -> (size(s)=w19:i32)
  n196 = case shown="2.." w19 {
    tunnel: w17 -> [_ w381]
    frame 0, Default {
    }
    frame 2.. {
      n197 = invoke class="VI" method="FP.Close"(error in=w381) -> ()  [unwired: 2 in, 3 out]
    }
  }
